vi "Simple_DAQ_AnalogIO.create DAQ channels.vi"(0 "i ref in":refnum<vi>, 1 "input_channels":string[](array[string]), 2 "output_channels":string[](array[string]), 3 "Timeout":i32=10000, 5 "error in":errorcluster caption="Fehler (Eingang, kein Fehler)") -> (14 "i ref out":refnum<vi>, 17 "timed out":bool, 19 "error out":errorcluster caption="Fehler (Ausgang)")   [LabVIEW 2014, in "Simple_DAQ_AnalogIO.lvlib"]
doc: "Contact: Falk Ziegler, eMail: info@lab-coding.de"
uses:
  Simple_DAQ_AnalogIO.lvlib
  <vilib>/DAQmx/create/channels.llb/DAQmx Create Channel (AO-Voltage-Basic).vi
  <vilib>/DAQmx/write.llb/DAQmx Write (Analog DBL 1Chan 1Samp).vi
  <vilib>/DAQmx/create/channels.llb/DAQmx Create Channel (AI-Voltage-Basic).vi
  CS_Core/CSSystem/CSSystemLib/CSSystemLib.lvlib
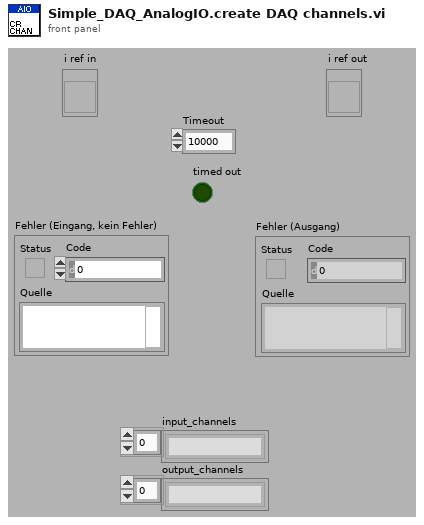
[diagram p1: front panel]
types:
  T1 = typedef "Simple_DAQ_AnalogIO.lvlib/Simple_DAQ_AnalogIO.i attribute.ctl" = cluster{"inputs":cluster{"index":i32[], "channel_task":refnum<k21>[], "range":cluster{"min":dbl, "max":dbl}[], "channel_number":i32, "scale_factor":dbl}, "outputs":cluster{"index":i32[], "channel_task":refnum<k21>[], "range":cluster{"min":dbl, "max":dbl}[], "channel_number":i32, "scale_factor":dbl}}
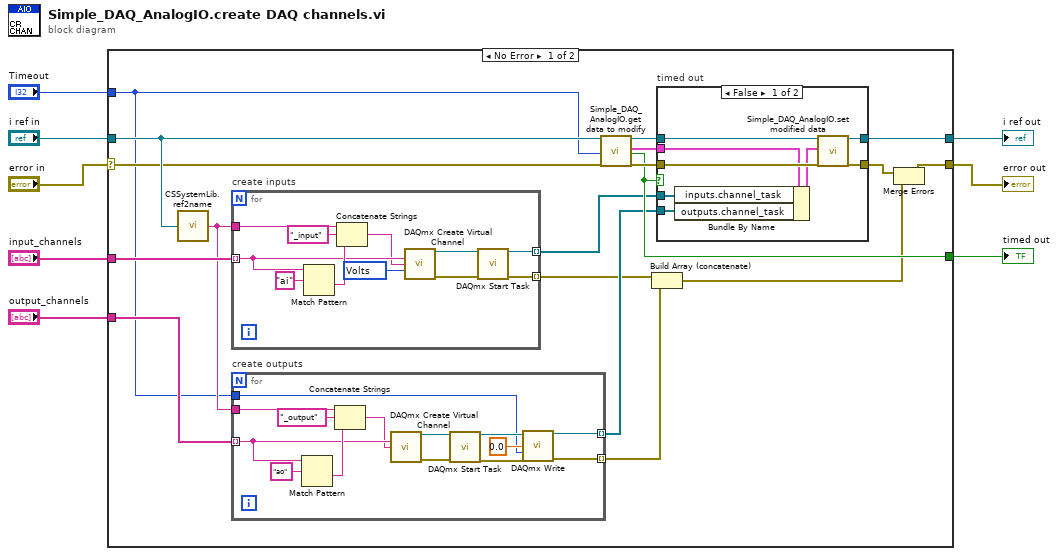
[diagram p0: block diagram]
diagram:
  n1 = case shown="No Error" "error in" {
    selector: "error in" -> [w23 w63]
    tunnel: "i ref in" -> [w24 w62]
    tunnel: [w16 w63] -> w6
    tunnel: [w20 w62] -> w5
    tunnel: "Timeout" -> [w13 _]
    tunnel: "input_channels" -> [w26 _]
    tunnel: "output_channels" -> [w15 _]
    tunnel: [w18 _] -> w1
    frame No Error {
      n2 = call "CSSystemLib.ref2name.vi"("obj refnum"=w24) -> ("name"=w25:string)
      n3 = for "create inputs" {
        tunnel: w26 -> [w41] mode=indexing
        tunnel: w25 -> [w44]
        tunnel: [w39] -> w11 mode=indexing
        tunnel: [w38] -> w14 mode=indexing
        w37 = 10348 items=["Volts"=10348, "From Custom Scale"=10065] ("units")
        n4 = Match Pattern(string=w41, regular expression="ai" ("regulärer Ausdruck")) -> (after substring=w47:string)  [unwired: 1 in, 3 out]
        n5 = Concatenate Strings(w44, "_input" ("String"), w47) -> (w40:string)
        n6 = call-poly <vilib>:"DAQmx Create Virtual Channel.vi"("physical channels"=w41, "name to assign"=w40, "units"=w37) -> ("task out"=w42:refnum<k21>, "error out"=w43:errorcluster)  [unwired: 11 in]
        n7 = call <vilib>:"DAQmx Start Task.vi"("task/channels in"=w42, "error in"=w43) -> ("task out"=w38:refnum<k21>, "error out"=w39:errorcluster)  [unwired: 12 in]
      }
      n8 = for "create outputs" {
        tunnel: w25 -> [w61]
        tunnel: w15 -> [w57] mode=indexing
        tunnel: [w54] -> w12 mode=indexing
        tunnel: w13 -> [w49]
        tunnel: [w50] -> w10 mode=indexing
        n9 = Match Pattern(string=w57, regular expression="ao" ("regulärer Ausdruck")) -> (after substring=w58:string)  [unwired: 1 in, 3 out]
        n10 = Concatenate Strings(w61, "_output" ("String"), w58) -> (w48:string)
        n11 = call-poly <vilib>:"DAQmx Create Virtual Channel.vi"("physical channels"=w57, "name to assign"=w48) -> ("task out"=w56:refnum<k21>, "error out"=w52:errorcluster)  [unwired: 12 in]
        n12 = call <vilib>:"DAQmx Start Task.vi"("task/channels in"=w56, "error in"=w52) -> ("task out"=w55:refnum<k21>, "error out"=w51:errorcluster)  [unwired: 12 in]
        n13 = call-poly <vilib>:"DAQmx Write.vi"("task/channels in"=w55, "data"=0.0, "timeout"=w49, "error in"=w51) -> ("task out"=w54:refnum<k21>, "error out"=w50:errorcluster)  [unwired: 9 in, 1 out]
      }
      n14 = call "Simple_DAQ_AnalogIO.get data to modify.vi"("i ref in"=w24, "ms timeout (10000)"=w13, "error in (no error)"=w23) -> ("i ref out"=w22:refnum<vi>, "i attribute"=w19:T1, "timed out"=w18:bool, "error out"=w21:errorcluster)  [unwired: 13 in]
      n15 = Build Array (concatenate)(w11, w10) -> (w9:errorcluster[])
      n16 = case "timed out" shown="False" w18 {
        tunnel: w22 -> [w32 w36]
        tunnel: w21 -> [w31 w35]
        tunnel: [w34 w36] -> w20
        tunnel: [w33 w35] -> w17
        tunnel: w19 -> [w30 _]
        tunnel: w14 -> [w28 _]
        tunnel: w12 -> [w27 _]
        frame False {
          n17 = Bundle By Name(cluster=w30, "inputs.channel_task"=w28, "outputs.channel_task"=w27) -> (w29:T1)
          n18 = call "Simple_DAQ_AnalogIO.set modified data.vi"("i ref in"=w32, "i attribute"=w29, "error in (no error)"=w31) -> ("i ref out"=w34:refnum<vi>, "error out"=w33:errorcluster)  [unwired: 15 in]
        }
        frame True {
        }
      }
      n19 = Merge Errors(w17, w9) -> (w16:errorcluster)
    }
    frame Error {
    }
  }
  "error out" <- w6
  "timed out" <- w1
  "i ref out" <- w5
